vi "Send ON Command.vi"(8 "error in (no error)":errorcluster) -> (0 "error out":errorcluster)   [LabVIEW 2014]
doc: "Sends the ON command to the myRIO. This tells the myRIO to turn the switch on."
uses:
  Controls/UDP Reference Action Enum.ctl
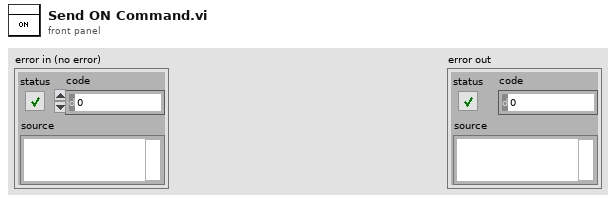
[diagram p1: front panel]
types:
  T1 = typedef "UDP Reference Action Enum.ctl" = enum16{"Set", "Get"}
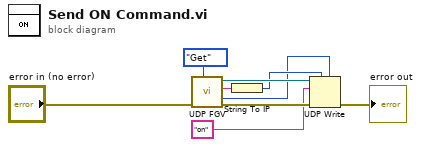
[diagram p0: block diagram]
diagram:
  n1 = call "UDP FGV.vi"("Action"=UDP_Reference_Action_Enum."Get", "error in (no error)"="error in (no error)") -> ("error out"=w7:errorcluster, "Port Out"=w2:u16, "IP Address out"=w4:string, "connection ID out"=w8:refnum<k16>)  [unwired: 6 in]
  n2 = String To IP(1:w4) -> (0:w3:u32)
  n3 = UDP Write(address=w3, port or service name=w2, connection ID=w8, data in="on", 8:w7) -> (error out=→"error out":errorcluster)  [unwired: 1 in, 1 out]
